vi "CLD 1 Elapsed Time Express Front Panel.vi"() -> ()   [LabVIEW 2025]
doc: "LabVIEW CLD 1 Exercise"
panel:
  out "error out":errorcluster
  in  "error in":errorcluster
  out "Elapsed Time":string
  out "Time has Elapsed":bool
  in  "Auto Reset":bool=TRUE
  in  "Reset Button":bool
  in  "Stop VI":bool
  in  "Time Target (s)":dbl=2.0
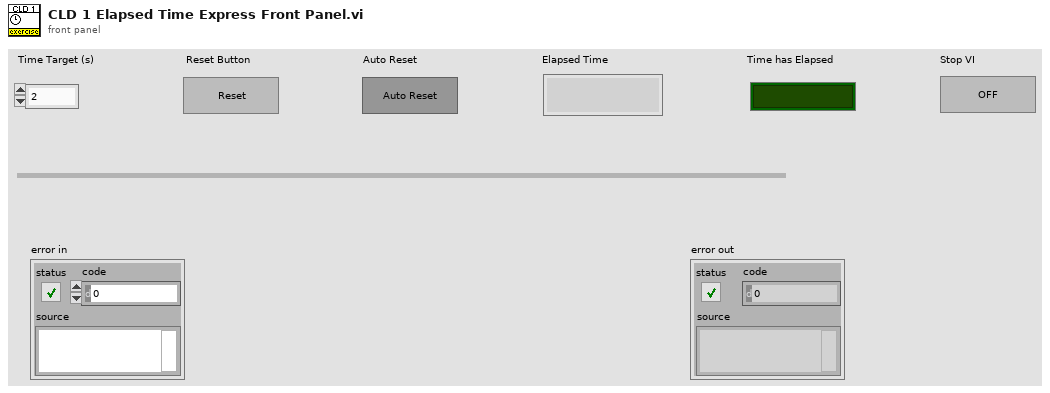
[diagram p1: front panel]
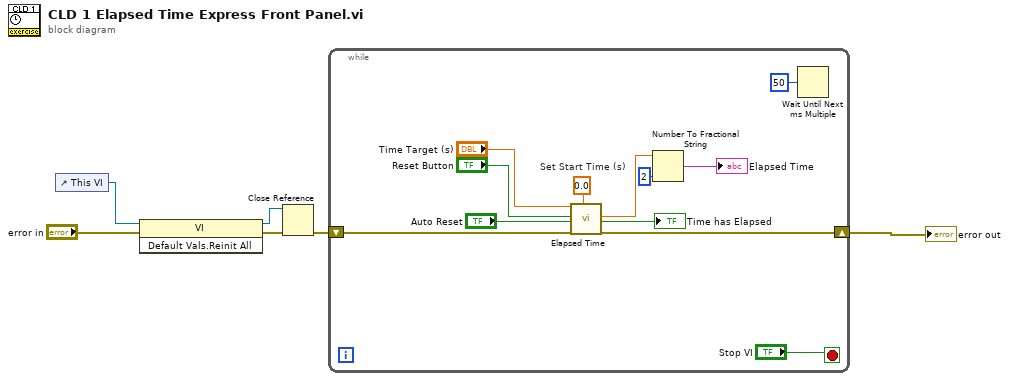
[diagram p0: block diagram]
diagram:
  n1 = control-ref of="This VI"() -> (w3:refnum<vi>)
  n2 = invoke class="VI" method="Default Vals.Reinit All"(reference=w3, error in="error in") -> (reference out=w1:refnum<vi>, error out=w4:errorcluster)  [unwired: 1 in, 1 out]
  n3 = Close Reference(reference=w1, error in (no error)=w4) -> (error out=w2:errorcluster)
  n4 = while {
    shift-right: [w17] -> w5
    shift-left: w2 -> [w18]
    stop <- "Stop VI" stop-if-true
    w14 = 0.0  # Set Start Time (s)
    n5 = call "Elapsed Time"("Time Target (s)"="Time Target (s)", "Reset"="Reset Button", "Auto Reset"="Auto Reset", "error in (no error)"=w18, "Set Start Time (s)"=w14) -> ("Elapsed Time (s)"=w11:dbl, "Time has Elapsed"=→"Time has Elapsed":bool, "error out"=w17:errorcluster)  [unwired: 7 in, 5 out]
    n6 = Number To Fractional String(number=w11, precision (6)=i16 2) -> (F-format string=→"Elapsed Time":string)  [unwired: 2 in]
    n7 = Wait Until Next ms Multiple(millisecond multiple=u32 50 ("milliseconds to wait")) -> ()  [unwired: 1 out]
  }
  "error out" <- w5
